vi "Get Plugin Paths.vi"(8 "error in":errorcluster, 11 "measurement plugin in":refnum<class "NI Switch Control.lvclass">) -> (0 "error out":errorcluster, 2 "plugin paths":T1, 3 "measurement plugin out":refnum<class "NI Switch Control.lvclass">)   [LabVIEW 2025, in "NI Switch Control.lvclass"]
uses:
  NI Switch Control.lvclass
  <vilib>/Plug-In SDKs/Measurements/Measurement Plugin Service/Plugin Paths.ctl
  Measurement Logic.vi
  Measurement Configuration.ctl
  Measurement Results.ctl
  <vilib>/Plug-In SDKs/Measurements/Measurement Plugin Service/Measurement Plugin Service.lvclass
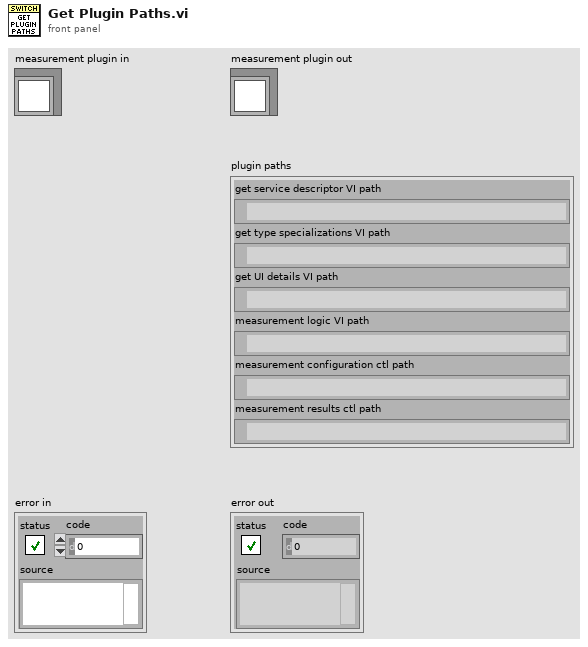
[diagram p1: front panel]
types:
  T1 = typedef "NI Measurement Plug-In SDK.lvlib/Measurement Plugin Service.lvclass/Plugin Paths.ctl" = cluster{"get service descriptor VI path":path, "get type specializations VI path":path, "get UI details VI path":path, "measurement logic VI path":path, "measurement configuration ctl path":path, "measurement results ctl path":path}
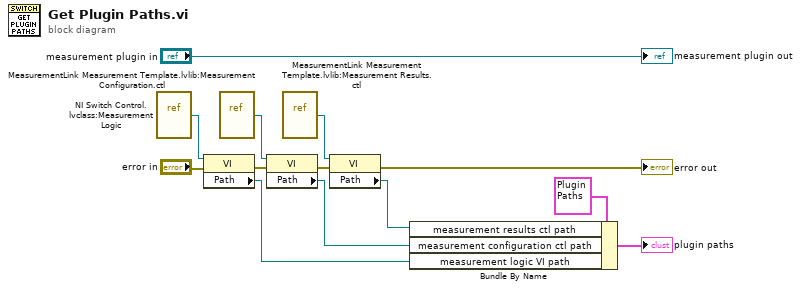
[diagram p0: block diagram]
diagram:
  n1 = vi-ref "NI Switch Control.lvclass:Measurement Logic.vi"() -> (w12:refnum<vi>)
  n2 = property class="VI"(reference=w12, error in="error in") -> (error out=w2:errorcluster, "Path"=w5:path)  [unwired: 1 out]
  n3 = vi-ref "MeasurementLink Measurement Template.lvlib:Measurement Configuration.ctl"() -> (w11:refnum<vi>)
  n4 = property class="VI"(reference=w11, error in=w2) -> (error out=w9:errorcluster, "Path"=w4:path)  [unwired: 1 out]
  n5 = vi-ref "MeasurementLink Measurement Template.lvlib:Measurement Results.ctl"() -> (w10:refnum<vi>)
  n6 = property class="VI"(reference=w10, error in=w9) -> (error out=→"error out":errorcluster, "Path"=w3:path)  [unwired: 1 out]
  n7 = Bundle By Name(cluster=T1 {"get service descriptor VI path"=path "", "get type specializations VI path"=path "", "get UI details VI path"=path "", "measurement logic VI path"=path "", "measurement configuration ctl path"=path "", "measurement results ctl path"=path ""} ("Plugin Paths"), "measurement results ctl path"=w3, "measurement configuration ctl path"=w4, "measurement logic VI path"=w5) -> (→"plugin paths":T1)
  "measurement plugin out" <- "measurement plugin in"
